vi "Visible3DArray.vi"(7 "Visible":bool=TRUE, 11 "Array In":cluster{"X":dbl[], "Y":dbl[], "Z":dbl[]}[](array[cluster])) -> (3 "Array Out":cluster{"X":dbl[], "Y":dbl[], "Z":dbl[]}[](array[cluster]))   [LabVIEW 2020]
doc: "Makes part of the data visible or invisible"
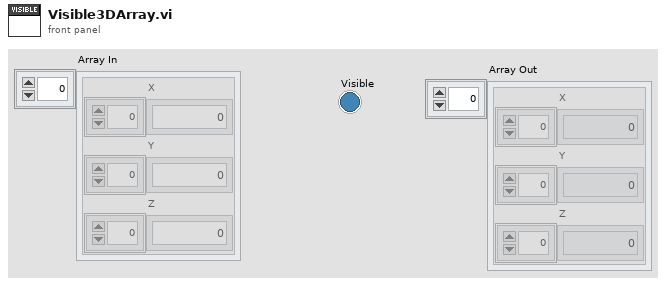
[diagram p1: front panel]
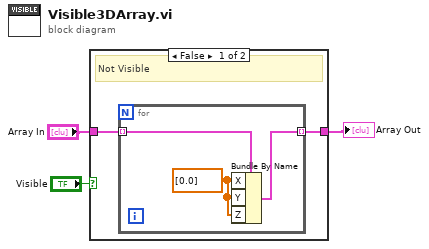
[diagram p0: block diagram]
diagram:
  n1 = case shown="False" "Visible" {
    tunnel: "Array In" -> [w5 w9]
    tunnel: [w4 w9] -> w1
    frame False {
      # "Not Visible"
      n2 = for {
        tunnel: w5 -> [w8] mode=indexing
        tunnel: [w7] -> w4 mode=indexing
        w6 = dbl[] [0.0] ("X")
        n3 = Bundle By Name(cluster=w8, "X"=w6, "Y"=w6, "Z"=w6) -> (w7:cluster{"X":dbl[], "Y":dbl[], "Z":dbl[]})
      }
    }
    frame True {
      # "Visible"
    }
  }
  "Array Out" <- w1
